vi "ABResistancePlotter.vi"() -> ()   [LabVIEW 2021]
panel:
  in  "milliseconds to wait":u32=10000
  out "Resistance":cluster{dbl, dbl}[](graph)
  out "Allen Bradley \nResistance":dbl format="%#_6p"
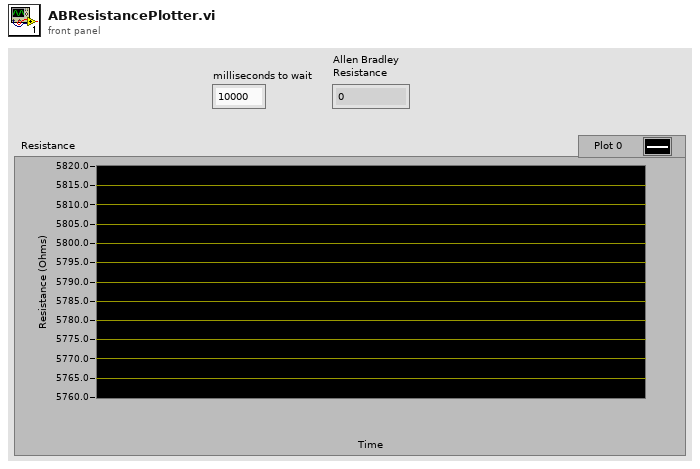
[diagram p1: front panel]
types:
  T1 = enum16{"Set Voltage", "Read Voltage", "Read Setpoint", "Read Current", "Output On", "Output Off"}
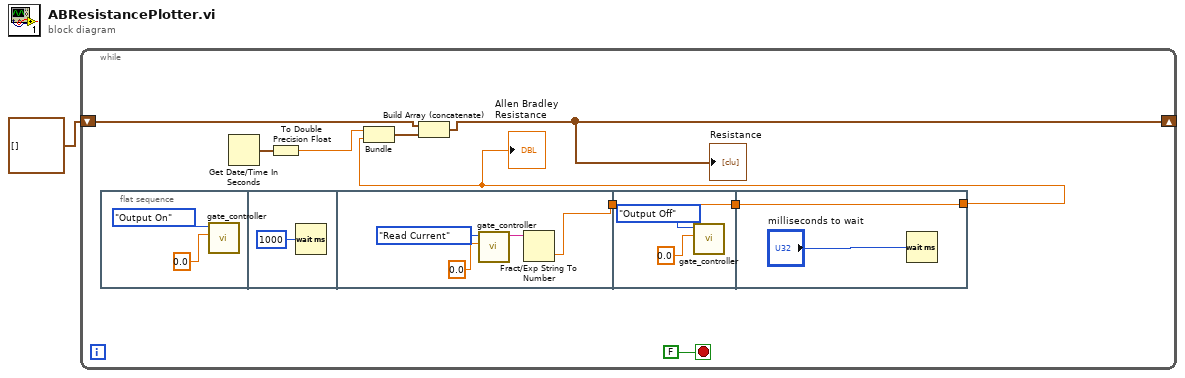
[diagram p0: block diagram]
diagram:
  n1 = while {
    shift-right: [w4] -> _
    shift-left: cluster{dbl, dbl}[] [] -> [w5]
    stop <- FALSE stop-if-true
    n2 = flat-sequence {
      tunnel: [w14] -> w3
      tunnel: w3 -> [w20]
      tunnel: [w20] -> w2
      tunnel: [w22] -> w7
      tunnel: w2 -> [w22]
      frame #0 {
        n3 = call "gate_controller.vi"("Numerical Argument"=0.0, "Command"=T1."Output On") -> ()  [unwired: 9 in, 1 out]
      }
      frame #1 {
        n4 = Wait (ms)(milliseconds to wait=u32 1000) -> ()  [unwired: 1 out]
      }
      frame #2 {
        n5 = call "gate_controller.vi"("Numerical Argument"=0.0, "Command"=T1."Read Current") -> ("Response"=w15:string)  [unwired: 9 in]
        n6 = Fract/Exp String To Number(string=w15) -> (number=w14:dbl)  [unwired: 3 in, 1 out]
      }
      frame #3 {
        n7 = call "gate_controller.vi"("Numerical Argument"=0.0, "Command"=T1."Output Off") -> ()  [unwired: 9 in, 1 out]
      }
      frame #4 {
        n8 = Wait (ms)(milliseconds to wait="milliseconds to wait") -> ()  [unwired: 1 out]
      }
    }
    n9 = Get Date/Time In Seconds() -> (seconds since 1Jan1904=w9:timestamp)
    n10 = To Double Precision Float(number=w9) -> (double precision float=w8:dbl)
    n11 = Bundle(w8, w7) -> (w6:cluster{dbl, dbl})  [unwired: 1 in]
    n12 = Build Array (concatenate)(w5, w6) -> (w4:cluster{dbl, dbl}[])
    "Resistance" <- w4
    "Allen Bradley \nResistance" <- w7
  }
